vi "ROI entry screen-Generate user menu.vi"(11 "Functional Viewer Menu in":refnum<k9>) -> (0 "error out":errorcluster, 3 "Functional Viewer Menu":refnum<k9>)   [LabVIEW 2017]
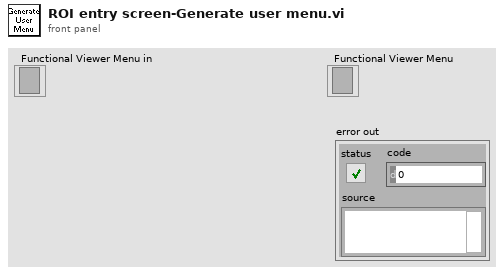
[diagram p1: front panel]
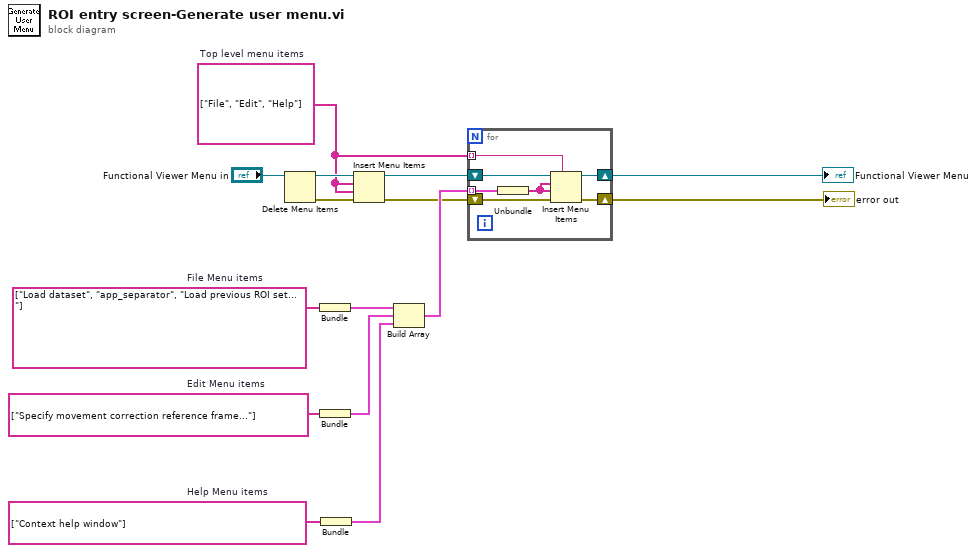
[diagram p0: block diagram]
diagram:
  w7 = string[] ["Context help window"]  # Help Menu items
  w8 = string[] ["Specify movement correction reference frame..."]  # Edit Menu items
  w10 = string[] ["Load dataset", "app_separator", "Load previous ROI set..."]  # File Menu items
  w11 = string[] ["File", "Edit", "Help"]  # Top level menu items
  n1 = Delete Menu Items(9:"Functional Viewer Menu in") -> (0:w15:errorcluster, 3:w14:refnum<k9>)  [unwired: 3 in]
  n2 = Bundle("File Menu items"=w10) -> (w9:cluster{"File Menu items":string[]})  [unwired: 1 in]
  n3 = Bundle("Edit Menu items"=w8) -> (w2:cluster{"Edit Menu items":string[]})  [unwired: 1 in]
  n4 = Bundle("Help Menu items"=w7) -> (w1:cluster{"Help Menu items":string[]})  [unwired: 1 in]
  n5 = Insert Menu Items(6:w15, 7:w11, 8:w11, 9:w14) -> (0:w3:errorcluster, 3:w12:refnum<k9>)  [unwired: 2 in, 1 out]
  n6 = Build Array(w9, w2, w1) -> (w6:cluster{"Help Menu items":string[]}[])
  n7 = for {
    shift-right: [w21] -> w5
    shift-left: w12 -> [w22]
    tunnel: w11 -> [w20] mode=indexing
    tunnel: w6 -> [w19] mode=indexing
    shift-right: [w17] -> w4
    shift-left: w3 -> [w16]
    n8 = Unbundle(w19) -> ("Help Menu items"=w18:string[])
    n9 = Insert Menu Items(5:w20, 6:w16, 7:w18, 8:w18, 9:w22) -> (0:w17:errorcluster, 3:w21:refnum<k9>)  [unwired: 1 in, 1 out]
  }
  "error out" <- w4
  "Functional Viewer Menu" <- w5
